vi "Discharge Prompt.vi"() -> (4 "output cluster":T1, 10 "Warm-Up":dbl, 14 "Cluster":T5, 15 "Cluster 2":T2)   [LabVIEW 2012]
panel:
  in  "Cut-Off Voltage":dbl
  in  "A Sensor Ratio(mV/A) (10.0000)":dbl=1.0 min=0.0001 max=99999.9999 step=0.0001 format="%.4f"
  in  "Wiring A (0: 1P2W)":enum16{"1P2W", "1P3W", "3P3W", "3P4W", "3V3A"}(ring)
  in  "A Range (9: 5A)":T3(ring)=enum."5 A"
  in  "V Range (12: 1000)":T4(ring)=enum."1000"
  in  "Warm-Up":dbl format="%<%H:%M:%S>t"
  in  "% Depth Of Discharge":dbl
  in  "Amp-Hours":dbl
  in  "Notes":string
  in  "Model":string
  in  "Manufactuere":string
  in  "Project":string
  in  "stop":bool
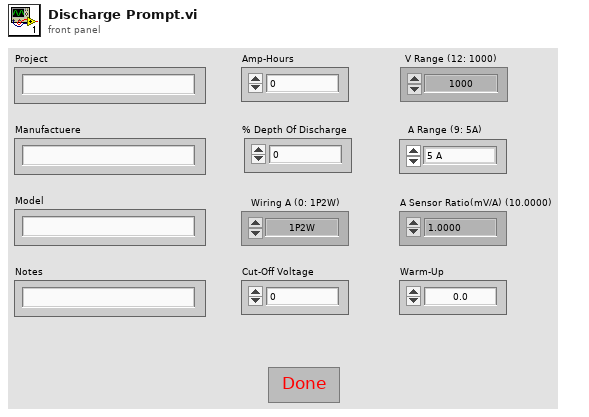
[diagram p1: front panel]
types:
  T1 = cluster{"Amp-Hours":dbl, "% Depth Of Discharge":dbl, "Cut-Off Voltage":dbl}
  T2 = cluster{"V Range (12: 1000)":u16, "A Range (9: 5A)":u16, "A Sensor Ratio(mV/A) (10.0000) ":dbl, "Wiring A (0: 1P2W)":u16}
  T3 = enum16{"AUTO", "10 mA", "20 mA", "50 mA", "100 mA", "200 mA", "500 mA", "1 A", "2 A", "5 A", "10 A", "20 A", "50 A", "S-AUTO", "50 mV", "100 mV", "250 mV", "500 mV", "1 V", "2.5 V", "5 V", "10 V"}
  T4 = enum16{"AUTO", "1.5", "3", "6", "10", "15", "30", "60", "100", "150", "300", "600", "1000"}
  T5 = cluster{"Project":string, "Manufactuere":string, "Model":string, "Notes":string}
  T6 = cluster{"V Range (12: 1000)":enum16{"AUTO", "1.5", "3", "6", "10", "15", "30", "60", "100", "150", "300", "600", "1000"}, "A Range (9: 5A)":enum16{"AUTO", "10 mA", "20 mA", "50 mA", "100 mA", "200 mA", "500 mA", "1 A", "2 A", "5 A", "10 A", "20 A", "50 A", "S-AUTO", "50 mV", "100 mV", "250 mV", "500 mV", "1 V", "2.5 V", "5 V", "10 V"}, "A Sensor Ratio(mV/A) (10.0000) ":dbl, "Wiring A (0: 1P2W)":enum16{"1P2W", "1P3W", "3P3W", "3P4W", "3V3A"}}
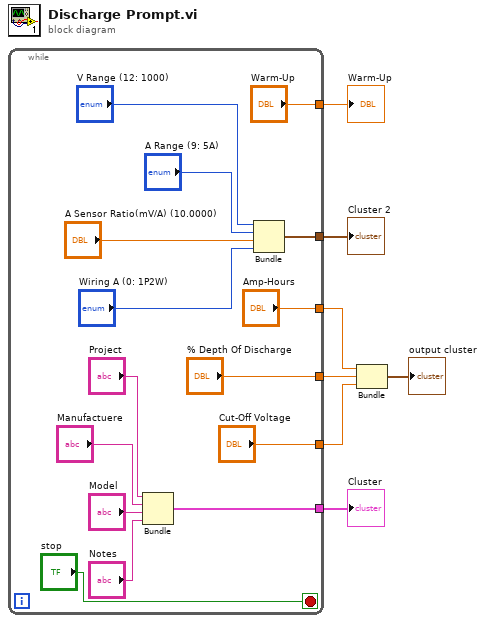
[diagram p0: block diagram]
diagram:
  n1 = while {
    tunnel: ["% Depth Of Discharge"] -> w3
    tunnel: ["Amp-Hours"] -> w4
    tunnel: [w15] -> w7
    tunnel: ["Warm-Up"] -> w6
    tunnel: [w11] -> w5
    tunnel: ["Cut-Off Voltage"] -> w2
    stop <- "stop" stop-if-true
    n2 = Bundle("Project"="Project", "Manufactuere"="Manufactuere", "Model"="Model", "Notes"="Notes") -> (w15:T5)  [unwired: 1 in]
    n3 = Bundle("V Range (12: 1000)"="V Range (12: 1000)", "A Range (9: 5A)"="A Range (9: 5A)", "A Sensor Ratio(mV/A) (10.0000)"="A Sensor Ratio(mV/A) (10.0000)", "Wiring A (0: 1P2W)"="Wiring A (0: 1P2W)") -> (w11:T6)  [unwired: 1 in]
  }
  "Cluster" <- w7
  "Warm-Up" <- w6
  "Cluster 2" <- w5
  n4 = Bundle("Amp-Hours"=w4, "% Depth Of Discharge"=w3, "Cut-Off Voltage"=w2) -> (→"output cluster":T1)  [unwired: 1 in]
